vi "Climb Controller.vi"(8 "error in":errorcluster) -> ()   [LabVIEW 2020]
doc: "This VI executes continuously carrying out the current operation and responding to updates or new operations. It will often contain the timing or control code that is difficult to place directly in TeleOp. This VI generally opens all sensors and motors and isolates the rest of the robot code from knowing how the operations are carried out."
uses:
  <vilib>/Rock Robotics/WPI/Framework/Completion Status.ctl
  Climb Setpoints.ctl
  Climb Operations.ctl
  <vilib>/Rock Robotics/WPI/SafetyOutput/WPI_SafetyOutputConfigMenu.ctl
  <vilib>/Rock Robotics/Network Tables/NT Write Number.vi
panel:
  in  "Interactive Values":T1
  out "Current\nCmd":string
  in  "Buttons":cluster{"Execute Cmd":bool, "Abort Cmd":bool}
  out "Command Timing":cluster{"Start Time (ms)":u32, "Iterations":i32}
  out "Status":T3
  # "Tip: It may be helpful to observe inputs and sensor values.\nYou may also want to display tuning or debugging controls."
  # "Interactive Command: You may fill in the settings for a command\nand schedule it with the Execute button. You can observe and abort\nany command while fine tuning the code for the controller."
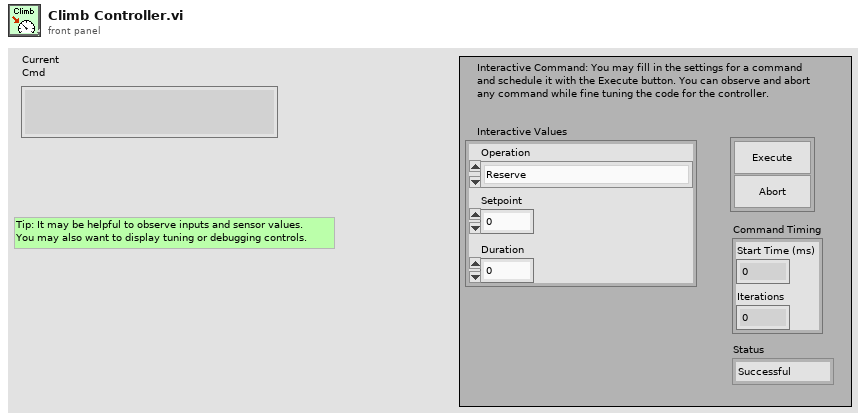
[diagram p1: front panel]
types:
  T1 = typedef "Climb Setpoints.ctl" = cluster{"Operation":T2, "Setpoint":dbl, "Duration":dbl}
  T2 = typedef "Climb Operations.ctl" = enum16{"Reserve", "Read Current", "Immediate", "For time", "Stop"}
  T3 = typedef "Completion Status.ctl" = enum16{"Successful", "Aborted", "Incomplete"}
  T4 = typedef "WPI_SafetyOutputConfigMenu.ctl" = enum16{"Enable", "Disable"}
  T5 = typedef "WPI_MotorControlDeviceRef.ctl" = cluster{"DeviceStatus":errorcluster, "Type":T6, "PWM":cluster{"PWM Channel":T7, "DeadBand":T8}, "CAN":cluster{"Device Number":u8, "SetOutput VI Ref":variant, "GetOutput VI Ref":variant, "Enable VI Ref":variant, "Disable VI Ref":variant, "Data":variant}, "Invert":bool, "DIO PWM":cluster{"PWM \"Enable\" Channel":T7, "DIOChannel":T9, "PWM Rate":dbl}}
  T6 = typedef "WPI_MotorControlType.ctl" = enum16{"PWM", "CAN", "DIO PWM"}
  T7 = typedef "FPGA_DIOPWMChannel.ctl" = enum8{"PWM 0", "PWM 1", "PWM 2", "PWM 3", "PWM 4", "PWM 5", "PWM 6", "PWM 7", "PWM 8", "PWM 9", "PWM MXP 0", "PWM MXP 1", "PWM MXP 2", "PWM MXP 3", "PWM MXP 4", "PWM MXP 5", "PWM MXP 6", "PWM MXP 7", "PWM MXP 8", "PWM MXP 9", "Invalid"}
  T8 = typedef "WPI_PWMDeadband.ctl" = cluster{"Name":string, "maxPositivePwm":i32, "minPositivePwm":i32, "centerPwm":i32, "maxNegativePwm":i32, "minNegativePwm":i32, "angularRange":u16}
  T9 = typedef "FPGA_DIOChannel.ctl" = enum8{"DIO 0", "DIO 1", "DIO 2", "DIO 3", "DIO 4", "DIO 5", "DIO 6", "DIO 7", "DIO 8", "DIO 9", "DIO MXP 0", "DIO MXP 1", "DIO MXP 2", "DIO MXP 3", "DIO MXP 4", "DIO MXP 5", "DIO MXP 6", "DIO MXP 7", "DIO MXP 8", "DIO MXP 9", "DIO MXP 10", "DIO MXP 11", "DIO MXP 12", "DIO MXP 13", "DIO MXP 14", "DIO MXP 15", "SPI Port CS1", "SPI Port CS2", "SPI Port CS3", "SPI Port MISO", "SPI Port MOSI", "Invalid"}
  T10 = typedef "Command Status Info.ctl" = cluster{"Name":string, "Status":T3, "notifier out":T11}
  T11 = typedef "Completion Notifier.ctl" = refnum<notifier>
  T12 = cluster{"Current Command":T1, "Command Timing":cluster{"Start Time (ms)":u32, "Iterations":i32}, "Command Arguments":cluster{"Command Info":T10, "Description":string, "Default Command":T1, "queue out":refnum<queue>, "Subsystem Name":string}}
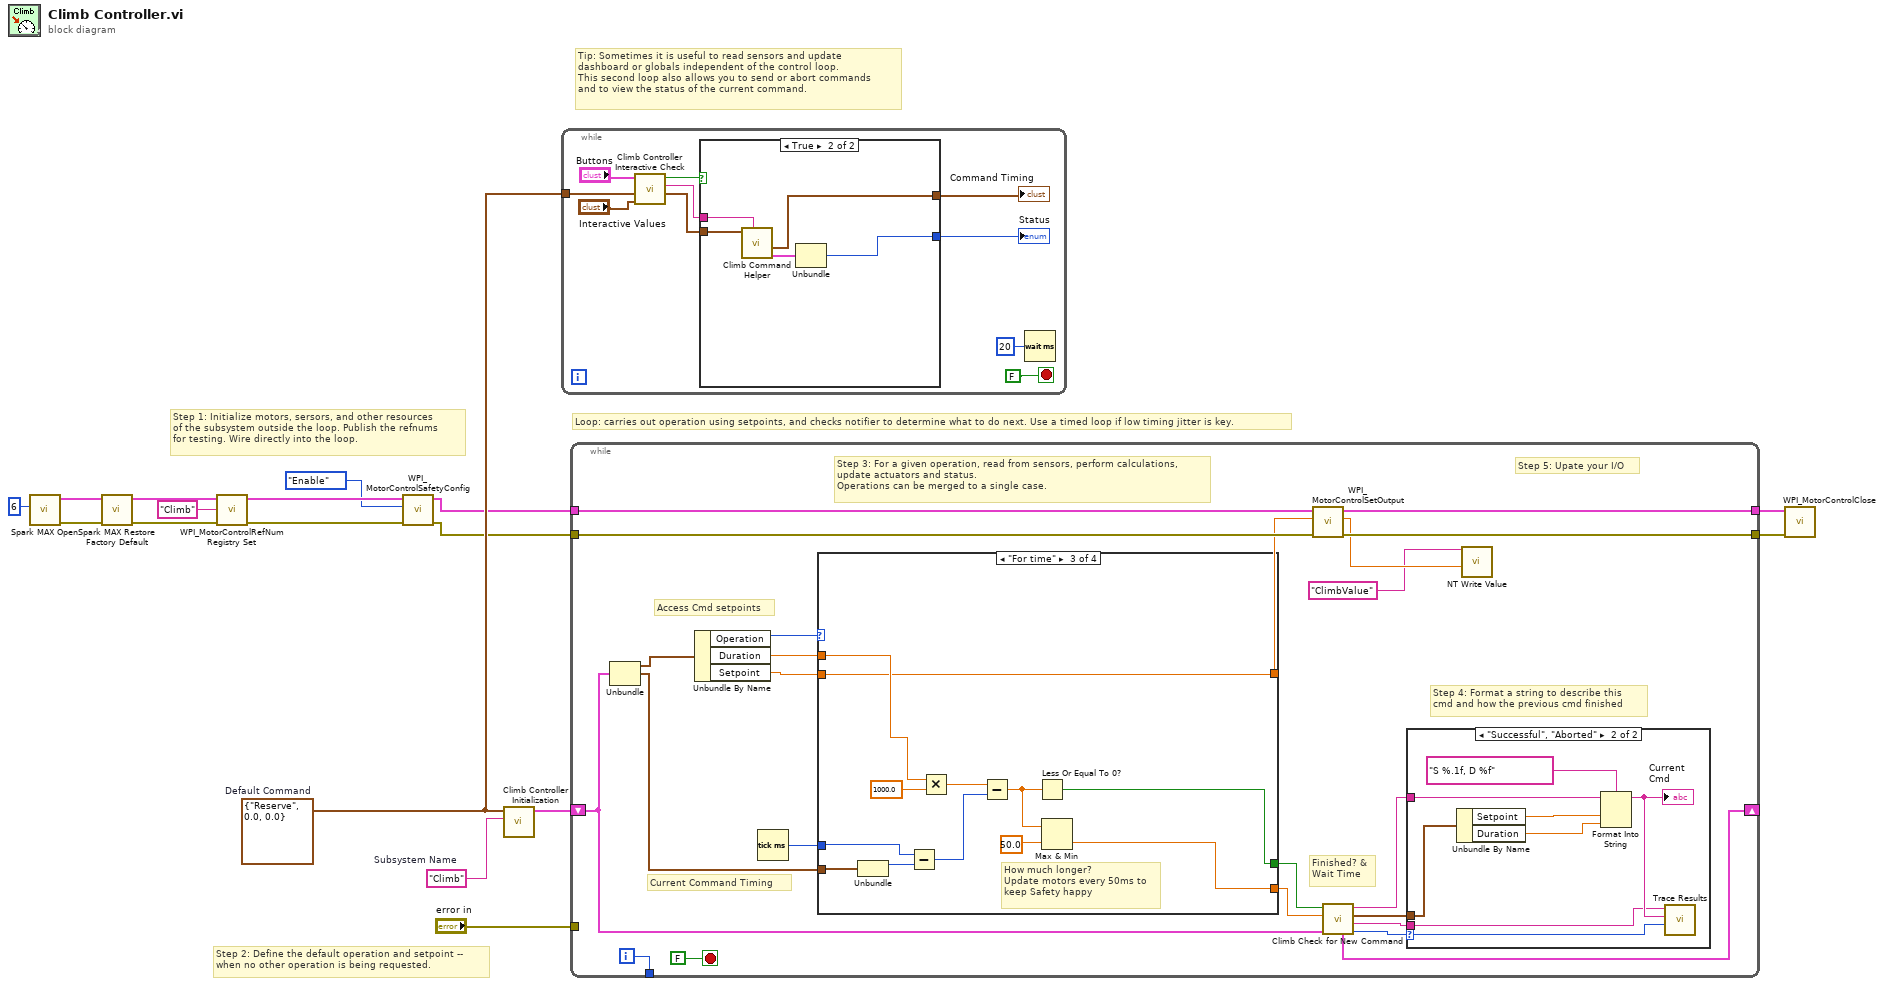
[diagram p0: block diagram]
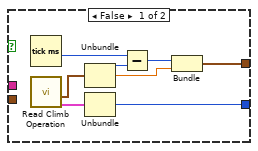
[diagram p2: hidden frame]
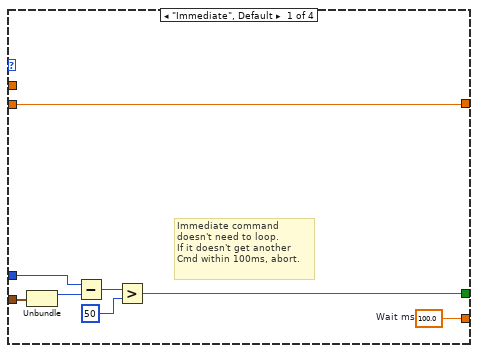
[diagram p4: hidden frame]
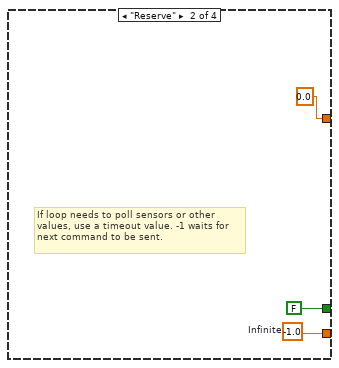
[diagram p5: hidden frame]
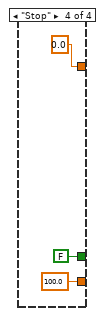
[diagram p6: hidden frame]
diagram:
  w14 = T1 {"Operation"=enum."Reserve", "Setpoint"=0.0, "Duration"=0.0}  # Default Command
  w15 = "Climb"  # Subsystem Name
  # "Tip: Sometimes it is useful to read sensors and update\ndashboard or globals independent of the control loop.\nThis second loop also allows you to send or abort commands\nand to view the status of the current command."
  # "Step 2: Define the default operation and setpoint --\nwhen no other operation is being requested."
  # "Step 1: Initialize motors, sersors, and other resources\nof the subsystem outside the loop. Publish the refnums\nfor testing. Wire directly into the loop."
  # "Loop: carries out operation using setpoints, and checks notifier to determine what to do next. Use a timed loop if low timing jitter is key."
  n1 = call <vilib>:"Spark MAX Open.vi"("Device Number"=u8 6) -> ("error out"=w13:errorcluster, "MotorControlDeviceRef"=w12:T5)  [unwired: 9 in]
  n2 = call <vilib>:"Spark MAX Restore Factory Default.vi"("error in"=w13, "MotorControlDeviceRef"=w12) -> ("error out"=w11:errorcluster, "MotorControlDeviceRef"=w10:T5)  [unwired: 8 in]
  n3 = call <vilib>:"WPI_MotorControlRefNum Registry Set.vi"("error in (no error)"=w11, "refnum name"="Climb", "MotorControlDevRef"=w10) -> ("error out"=w9:errorcluster, "MotorControlDevRef"=w8:T5)  [unwired: 7 in]
  n4 = call <vilib>:"WPI_MotorControlSafetyConfig.vi"("error in (no error)"=w9, "mode"=WPI_SafetyOutputConfigMenu."Enable", "MotorControlDevRef"=w8) -> ("error out"=w3:errorcluster, "MotorControlDevRef"=w4:T5)  [unwired: 7 in]
  n5 = call "Climb Controller Initialization.vi"("Subsystem Name"=w15, "Default Command"=w14) -> ("Current Command"=w16:T12)  [unwired: 9 in]
  n6 = while {
    tunnel: w14 -> [w24]
    stop <- FALSE stop-if-true
    n7 = call "Climb Controller Interactive Check.vi"("Interactive Command in"="Interactive Values", "Default Command"=w24, "Buttons"="Buttons") -> ("Interactive Command out"=w21:T1, "Trace String"=w22:string, "Schedule"=w23:bool)  [unwired: 6 in]
    n8 = case shown="True" w23 {
      tunnel: [w35 w40] -> w20
      tunnel: w21 -> [_ w38]
      tunnel: [w31 w36] -> w19
      tunnel: w22 -> [_ w39]
      frame False {
        n9 = Tick Count (ms)() -> (millisecond timer value=w30:u32)
        n10 = call "Read Climb Operation.vi"() -> ("Command Info"=w28:T10, "SubSystem Data"=w29:T1)  [unwired: 9 in, 1 out]
        n11 = Unbundle(w29) -> ("Operation"=w34:T2, "Setpoint"=w32:dbl)  [unwired: 1 out]
        n12 = Unbundle(w28) -> ("Status"=w35:T3)  [unwired: 2 out]
        n13 = Subtract(x=w30, y=w34) -> (x-y=w33:u32)
        n14 = Bundle(w33, "Setpoint"=w32) -> (w31:cluster{u32, "Setpoint":dbl})  [unwired: 1 in]
      }
      frame True {
        n15 = call "Climb Command Helper.vi"("Description"=w39, "SubSystem Data"=w38) -> ("Command Info Out"=w37:T10, "Command Timing"=w36:cluster{"Start Time (ms)":u32, "Iterations":i32})  [unwired: 7 in, 1 out]
        n16 = Unbundle(w37) -> ("Status"=w40:T3)  [unwired: 2 out]
      }
    }
    "Status" <- w20
    "Command Timing" <- w19
    n17 = Wait (ms)(milliseconds to wait=u32 20) -> ()  [unwired: 1 out]
  }
  n18 = while {
    shift-right: [w55] -> _
    shift-left: w16 -> [w48]
    tunnel: [w62] -> _
    tunnel: "error in" -> [_]
    tunnel: w4 -> [w47]
    tunnel: w3 -> [w46]
    tunnel: [w45] -> w2
    tunnel: [w44] -> w1
    i -> [w62]
    stop <- FALSE stop-if-true
    # "Step 5: Upate your I/O"
    # "Step 4: Format a string to describe this\ncmd and how the previous cmd finished"
    # "Current Command Timing"
    # "Access Cmd setpoints"
    # "Finished? &\nWait Time"
    # "Step 3: For a given operation, read from sensors, perform calculations,\nupdate actuators and status.\nOperations can be merged to a single case."
    n19 = Unbundle(w48) -> ("Current Command"=w61:T1, "Command Timing"=w57:cluster{"Start Time (ms)":u32, "Iterations":i32})  [unwired: 1 out]
    n20 = Unbundle By Name(w61) -> ("Operation"=w60:T2, "Duration"=w59:dbl, "Setpoint"=w56:dbl)
    n21 = Tick Count (ms)() -> (millisecond timer value=w58:u32)
    n22 = case shown="\"For time\"" w60 {
      tunnel: [w79 w82 w84 100.0 ("Infinite")] -> w53
      tunnel: [w73 FALSE ("ignore previous (F)") w85 FALSE ("ignore previous (F)")] -> w54
      tunnel: w57 -> [w75 _ w87 _]
      tunnel: w59 -> [_ _ w86 _]
      tunnel: w58 -> [w74 _ w88 _]
      tunnel: w56 -> [w72 _ w83 _]
      tunnel: [w72 0.0 ("Setpoint") w83 0.0 ("Setpoint")] -> w43
      frame "Immediate", Default {
        w79 = 100.0  # Wait ms
        # "Immediate command\ndoesn't need to loop.\nIf it doesn't get another\nCmd within 100ms, abort."
        n23 = Unbundle(w75) -> ("Start Time (ms)"=w78:u32)  [unwired: 1 out]
        n24 = Subtract(x=w74, y=w78) -> (x-y=w77:u32)
        n25 = Greater?(x=w77, y=u8 50 ("Left Motor")) -> (0:w73:bool)
      }
      frame "Reserve" {
        w82 = -1.0  # Infinite
        # "If loop needs to poll sensors or other\nvalues, use a timeout value. -1 waits for\nnext command to be sent."
      }
      frame "For time" {
        # "How much longer?\nUpdate motors every 50ms to\nkeep Safety happy"
        n26 = Unbundle(w87) -> ("Start Time (ms)"=w91:u32)  [unwired: 1 out]
        n27 = Subtract(x=w88, y=w91) -> (x-y=w94:u32)
        n28 = Multiply(x=w86, y=1000.0) -> (x*y=w93:dbl)
        n29 = Subtract(x=w93, y=w94) -> (x-y=w90:dbl)
        n30 = Less Or Equal To 0?(x=w90) -> (x <= 0?=w85:bool)
        n31 = Max & Min(x=w90, y=50.0) -> (min(x,y)=w84:dbl)  [unwired: 1 out]
      }
      frame "Stop" {
      }
    }
    n32 = call <vilib>:"WPI_MotorControlSetOutput.vi"("error in (no error)"=w46, "Output"=w43, "MotorControlDevRef"=w47) -> ("error out"=w44:errorcluster, "Motor Output"=w42:dbl, "MotorControlDevRef"=w45:T5)  [unwired: 6 in]
    n33 = call "Climb Check for New Command.vi"("Current Command"=w48, "Wait time (ms)"=w53, "Finished?"=w54) -> ("Completion"=w49:T3, "Subsystem Name"=w50:string, "Current Command"=w51:T1, "Initial Trace String"=w52:string, "NextCommand"=w55:T12)  [unwired: 4 in]
    n34 = case shown="\"Successful\", \"Aborted\"" w49 {
      selector: w49 -> [_ w71]
      tunnel: w52 -> [_ w67]
      tunnel: w51 -> [_ w68]
      tunnel: w50 -> [_ w64]
      frame "Incomplete", Default {
        # "Continuing current command"
      }
      frame "Successful", "Aborted" {
        # "Report and setup for next command"
        n35 = Unbundle By Name(w68) -> ("Setpoint"=w70:dbl, "Duration"=w65:dbl)
        n36 = Format Into String(format string="S %.1f, D %f", initial string=w67, w70, w65) -> (resulting string=w66:string)  [unwired: 1 in, 1 out]
        "Current\nCmd" <- w66
        n37 = call <vilib>:"Trace Results.vi"("Status of previous command"=w71, "Description"=w66, "Subsystem"=w64) -> ()  [unwired: 9 in]
      }
    }
    n38 = call-poly <vilib>:"NT Write Value.vi"("Numeric"=w42, "Name"="ClimbValue") -> ()  [unwired: 9 in, 1 out]
  }
  n39 = call <vilib>:"WPI_MotorControlClose.vi"("error in"=w1, "MotorControlDevRef"=w2) -> ()  [unwired: 9 in, 1 out]
